vi "Initialize S3DK.vi"(8 "error in (no error)":errorcluster, 11 "Settings IN":T1={"State"=enum."Idle S3DK", "Settings"="", "Online"=FALSE, "S3DK"={"Signals"={"Phasor"=[], "Analog"=[], "Digital"=[]}}, "CSV"={"Index"=0, "Parcel Length"=0, "EOF?"=FALSE, "Config"={"Mode"=enum."Full timestamp", "delimiter (\\t)"="\t", "Path"=path "", "Rectangular?"=FALSE}}}) -> (0 "error out":errorcluster, 3 "Settings OUT":T1={"State"=enum."Idle S3DK", "Settings"="", "Online"=FALSE, "S3DK"={"Signals"={"Phasor"=[], "Analog"=[], "Digital"=[]}}, "CSV"={"Index"=0, "Parcel Length"=0, "EOF?"=FALSE, "Config"={"Mode"=enum."Full timestamp", "delimiter (\\t)"="\t", "Path"=path "", "Rectangular?"=FALSE}}})   [LabVIEW 2017, in "Acquisition.lvlib"]
doc: "Initialize the hardware references."
uses:
  Acquisition.lvlib
  Acquisition Settings.ctl
  Acquisition State.ctl
  support/libs/CSV Reader/Mode CSV reader.ctl
  <vilib>/S3DK/PMU Recorder Light/PMU Recorder Light.lvlib
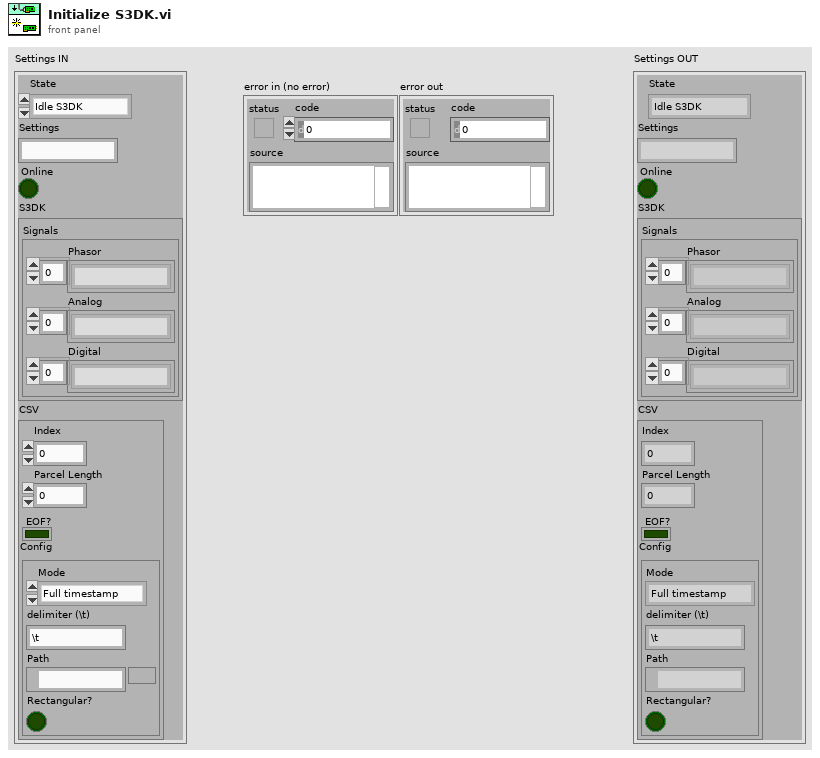
[diagram p1: front panel]
types:
  T1 = typedef "Acquisition.lvlib/Acquisition Settings.ctl" = cluster{"State":T2, "Settings":string, "Online":bool, "S3DK":cluster{"Signals":cluster{"Phasor":string[], "Analog":string[], "Digital":string[]}}, "CSV":cluster{"Index":i32, "Parcel Length":i32, "EOF?":bool, "Config":cluster{"Mode":T3, "delimiter (\\t)":string, "Path":path, "Rectangular?":bool}}}
  T2 = typedef "Acquisition.lvlib/Acquisition State.ctl" = enum16{"Idle", "Idle S3DK", "Acquiring S3DK", "Idle CSV", "Acquiring CSV"}
  T3 = typedef "Mode CSV reader.ctl" = enum16{"Full timestamp", "Relative Time", "Seconds Time", "Nanoseconds Time"}
  T4 = enum16{"Run", "Startup", "Get Status", "Pause", "Continue", "Shutdown", "Abort", "Open Panel", "Close Panel"}
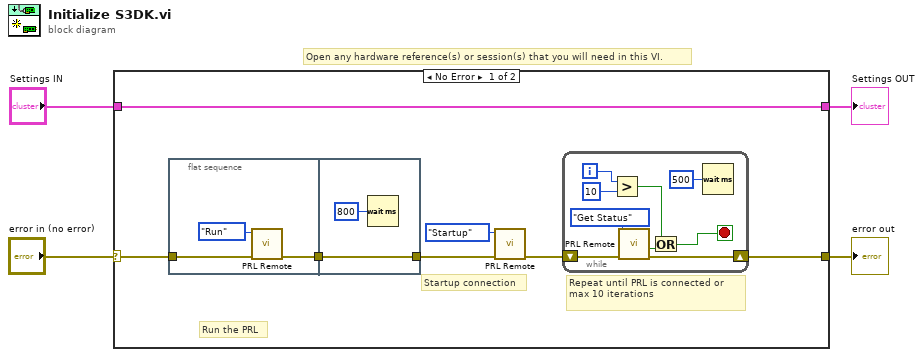
[diagram p0: block diagram]
diagram:
  # "Open any hardware reference(s) or session(s) that you will need in this VI."
  n1 = case shown="No Error" "error in (no error)" {
    selector: "error in (no error)" -> [w7 w26]
    tunnel: [w6 w26] -> w3
    tunnel: "Settings IN" -> [w11 w27]
    tunnel: [w11 w27] -> w1
    frame No Error {
      # "Run the PRL"
      # "Repeat until PRL is connected or max 10 iterations"
      # "Startup connection"
      n2 = flat-sequence {
        tunnel: w7 -> [w13]
        tunnel: [w14] -> w5
        tunnel: [w16] -> w9
        tunnel: w5 -> [w16]
        frame #0 {
          n3 = call <vilib>:"PRL Remote.vi"("error in (no error)"=w13, "Action"=T4."Run") -> ("error out"=w14:errorcluster)  [unwired: 4 in, 5 out]
        }
        frame #1 {
          n4 = Wait (ms)(milliseconds to wait=u32 800) -> ()  [unwired: 1 out]
        }
      }
      n5 = call <vilib>:"PRL Remote.vi"("error in (no error)"=w9, "Action"=T4."Startup") -> ("error out"=w10:errorcluster)  [unwired: 4 in, 5 out]
      n6 = while {
        shift-right: [w18] -> w6
        shift-left: w10 -> [w17]
        i -> [w23]
        stop <- w24 stop-if-true
        n7 = Greater?(x=w23, y=10) -> (0:w21:bool)
        n8 = call <vilib>:"PRL Remote.vi"("error in (no error)"=w17, "Action"=T4."Get Status") -> ("error out"=w18:errorcluster, "Connected"=w20:bool)  [unwired: 4 in, 4 out]
        n9 = Or(x=w21, y=w20) -> (x .or. y?=w24:bool)
        n10 = Wait (ms)(milliseconds to wait=u32 500) -> ()  [unwired: 1 out]
      }
    }
    frame Error {
    }
  }
  "Settings OUT" <- w1
  "error out" <- w3
